vi "DSF.Engine.Memory.Buffer.Write.1D.Bool.vi"(7 "count (-1: all)":i64=-1 format="%d elements", 8 "error in (no error)":errorcluster, 9 "offset (0)":u64 format="%d bytes", 10 "buffer in":bool[](array[boolean]), 11 "Buffer in":refnum<class "DSF.Engine.Memory.Buffer.lvclass">) -> (0 "error out":errorcluster, 1 "offset out":u64 format="%d bytes", 2 "buffer out":bool[](array[boolean]), 3 "Buffer out":refnum<class "DSF.Engine.Memory.Buffer.lvclass">)   [LabVIEW 2016, in "DSF.Engine.lvlib" / "DSF.Engine.Memory.Buffer.lvclass"]
uses:
  DSF.Engine.Memory.Buffer.lvclass
  C:/Git/Sourcetree/DSF/Source/Submodules/Memory/Source/Classes/Pointer/Memory.Pointer.lvclass
  Submodules/Memory/Source/Classes/Pointer/Memory.Pointer.lvclass/Memory.Pointer.ctl
  Submodules/Memory/Source/Classes/Pointer/Memory.Pointer.Write.Safe.1D.Bool.vi
  Submodules/Memory/Source/Classes/Pointer/Memory.Pointer.Write.Unsafe.1D.Bool.vi
  Submodules/Memory/Source/Classes/Pointer/Memory.Pointer.Parameter Check.Null Pointer.vi
  Submodules/Memory/Source/Classes/Pointer/Memory.Pointer.Parameter Check.Subset.Power of 2.vi
  Submodules/Memory/Source/Classes/Pointer/Memory.Pointer.Get Address.vi
  Submodules/Memory/Source/Classes/Pointer/Memory.Pointer.Errors.vi
  Submodules/Memory/Source/Classes/Pointer/Memory.Pointer.Errors.Null Pointer.vi
  Submodules/Memory/Source/Classes/Pointer/Memory.Pointer.Errors.Out of Bounds.vi
  Submodules/Memory/Source/Classes/Pointer/Memory.Pointer.Get Size.vi
  Submodules/Memory/Source/VIs/Memory.Count to Size.Power of 2.vi
  Submodules/Memory/Source/Classes/Pointer/Memory.Pointer.Errors.Create Error.vi
  Submodules/Memory/Source/Submodules/SEH/Source/VIs/Static Error Handling.Source Buffer.Write.String.vi
  Submodules/Memory/Source/Classes/Pointer/Memory.Pointer.Errors.Write Pointer Size.vi
  Submodules/Memory/Source/Submodules/SEH/Source/VIs/Static Error Handling.Source Buffer.Write.Numeric.Scalar.Base10.vi
  Submodules/Memory/Source/Submodules/SEH/Source/VIs/Static Error Handling.Source Buffer.Write.Numeric.Scalar.Base10 (U64).vi
  Submodules/Memory/Source/Submodules/SEH/Source/VIs/Static Error Handling.Error Cluster Constant.vi
  Submodules/Memory/Source/Submodules/SEH/Source/VIs/Static Error Handling.Error Cluster Constant (256B).vi
  Submodules/Memory/Source/Submodules/SEH/Source/VIs/Static Error Handling.Parameters.Status.Set.vi
  Submodules/Memory/Source/Submodules/SEH/Source/VIs/Static Error Handling.Parameters.Code.Set.vi
  Submodules/Memory/Source/Submodules/SEH/Source/VIs/Static Error Handling.Parameters.VI Source.Set.vi
  Submodules/Memory/Source/Constants/Memory.Constants.vi
  Submodules/Memory/Source/Constants/Memory.Constants.Library Name.vi
  Submodules/Memory/Source/Classes/Pointer/Memory.Pointer.Errors.Get Info.vi
  Submodules/Memory/Source/Classes/Pointer/Memory.Pointer.lvclass
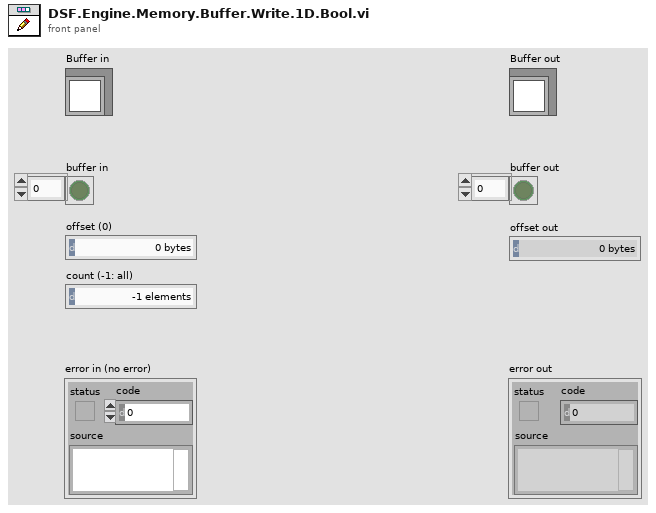
[diagram p1: front panel]
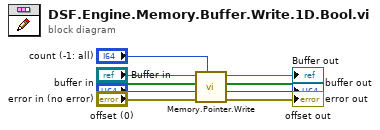
[diagram p0: block diagram]
diagram:
  n1 = call-poly "Memory.Pointer.Write.vi"("count (-1: all)"="count (-1: all)", "error in (no error)"="error in (no error)", "offset (0)"="offset (0)", "buffer in"="buffer in", "pointer in"="Buffer in") -> ("error out"=→"error out":errorcluster, "offset out"=→"offset out":u64, "buffer out"=→"buffer out":bool[], "pointer out"=→"Buffer out":refnum<class "DSF.Engine.Memory.Buffer.lvclass">)  [unwired: 3 in]
